vi "Numeric.vi"() -> ()   [LabVIEW 2023]
panel:
  out "time string 2":string
  out "String 2":string
  in  "Time Stamp":timestamp
  out "Numeric 3":dbl
  in  "Knob":dbl(knob) scale=0.0..10.0
  out "Numeric 2":dbl
  in  "Color Box":u32(colorbox)
  in  "Scrollbar 2":i32(c297)
  in  "Scrollbar":i32(c297)
  out "Thermometer":dbl(slide) scale=0.0..100.0
  out "Tank":dbl(slide) scale=0.0..10.0
  out "Gauge":dbl(knob) scale=0.0..10.0
  out "Meter":dbl(knob) scale=0.0..10.0
  in  "Dial":dbl(knob) scale=0.0..10.0
  out "Slide 6":u8(slide) scale=0.0..100.0
  in  "Slide 5":dbl(slide) scale=0.0..10.0
  in  "Slide 4":dbl(slide) scale=0.0..10.0
  out "Slide 3":u8(slide) scale=0.0..100.0
  in  "Slide 2":dbl(slide) scale=0.0..10.0
  in  "Slide":dbl(slide) scale=0.0..10.0
  out "Time Stamp 2":timestamp
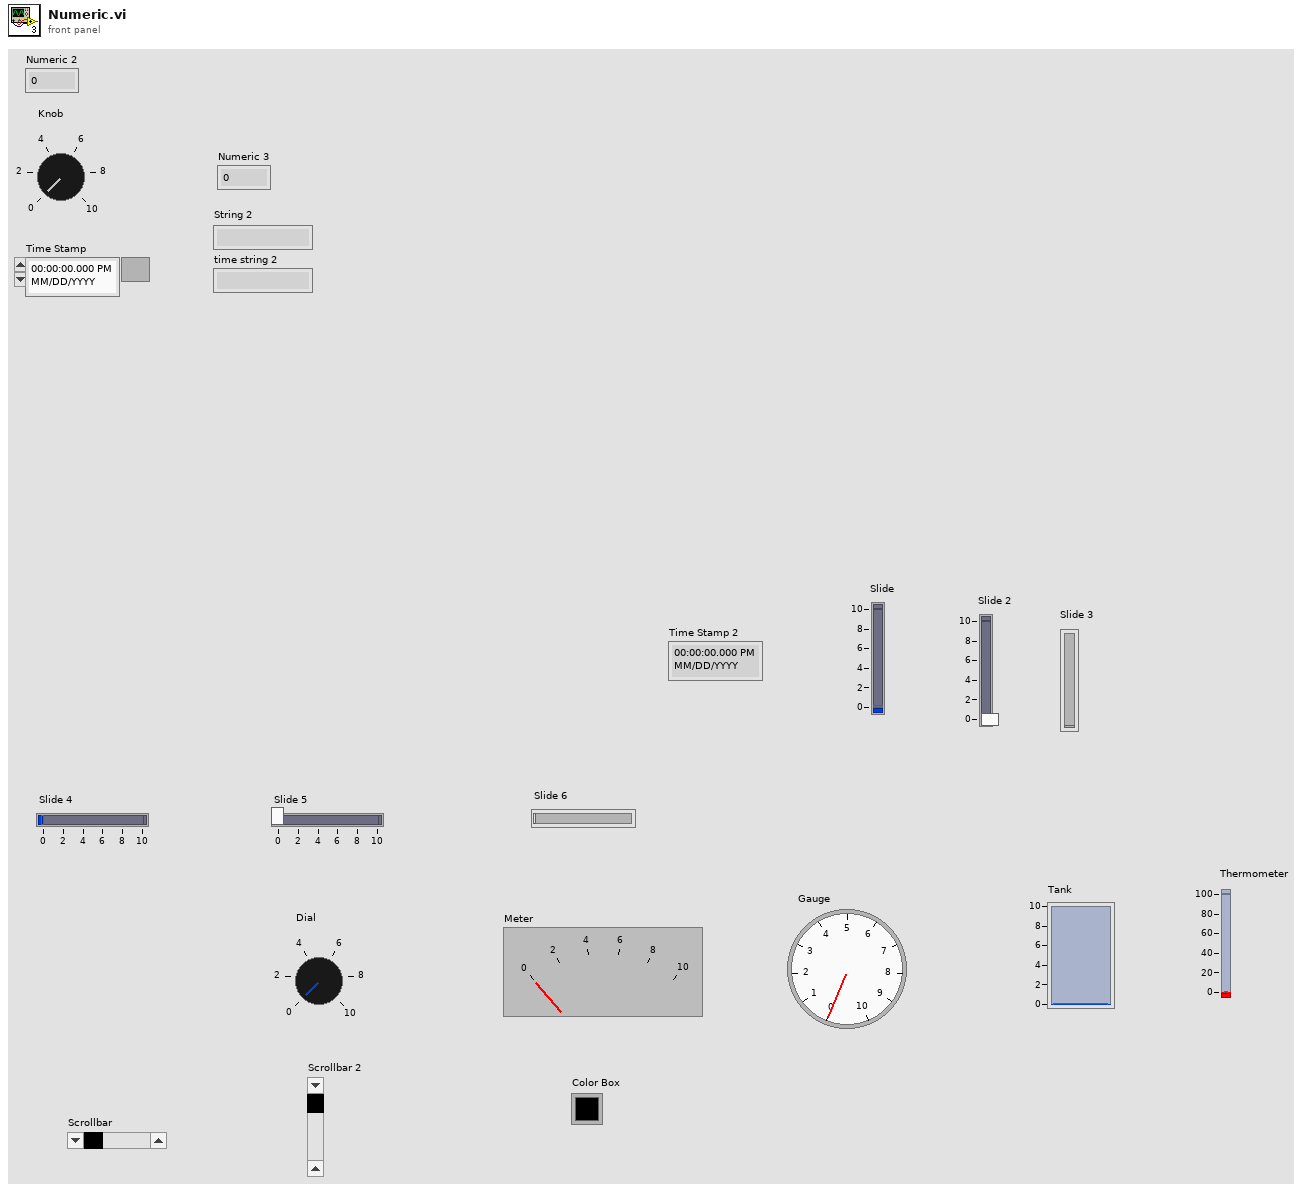
[diagram p1: front panel]
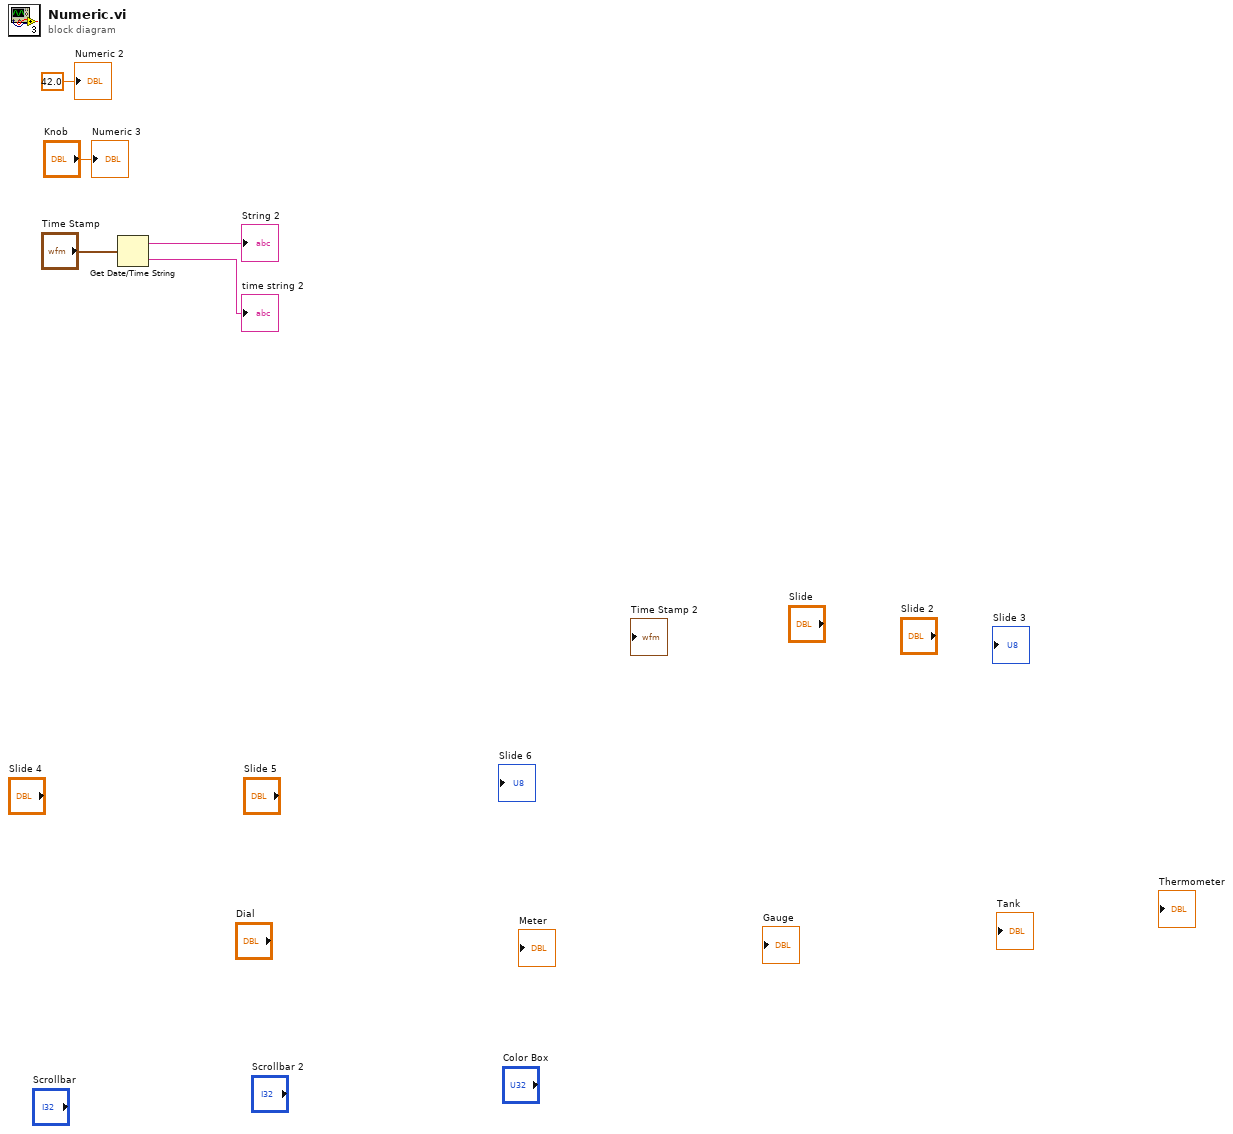
[diagram p0: block diagram]
diagram:
  n1 = Get Date/Time String(seconds (now)="Time Stamp") -> (date string=→"String 2":string, time string=→"time string 2":string)  [unwired: 2 in]
  "Numeric 2" <- 42.0 ("Numeric")
  "Numeric 3" <- "Knob"
